vi "Deinitialize.vi"(8 "error in":errorcluster, 11 "Channel":u16) -> (0 "error out":errorcluster)   [LabVIEW 2025, in "PCAN API.lvlib"]
doc: "This VI is used to deinitialize a CAN port."
uses:
  PCAN API.lvlib
  57794e42-bff5-43e6-b346-a6eef44ee780.vi
  PCAN2023/PCAN2023.lvlib
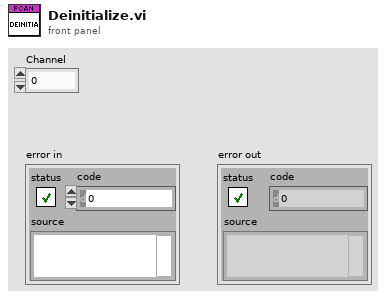
[diagram p1: front panel]
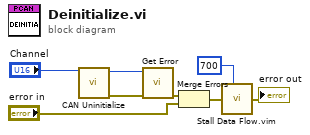
[diagram p0: block diagram]
diagram:
  n1 = call "CAN Uninitialize.vi"("Channel"="Channel") -> ("error out"=w7:errorcluster, "function return"=w5:u32)  [unwired: 9 in]
  n2 = call "Get Error.vi"("error in (no error)"=w7, "function return"=w5) -> ("error out"=w6:errorcluster)  [unwired: 9 in]
  n3 = Merge Errors(w6, "error in") -> (w4:errorcluster)
  n4 = call "Stall Data Flow.vim"("value in"=w4, "milliseconds to wait"=u32 700) -> ("value out"=→"error out":errorcluster)  [unwired: 1 out]
